vi "Create Plugins (old).vi"(5 "options":T1, 7 "framework configuration":T5, 8 "error in (no error)":errorcluster, 11 "Framework in":refnum<class "Framework.lvclass">) -> (0 "error out":errorcluster, 1 "Plugin Threads":refnum<class "Plugin Thread.lvclass">[](array[class]), 2 "Plugins":refnum<class "Plugin.lvclass">[](array[class]), 3 "Framework out":refnum<class "Framework.lvclass">)   [LabVIEW 2017, in "DSF Core.lvlib" / "Framework.lvclass"]
uses:
  Framework.lvclass
  Plugin/Plugin.lvclass
  DSF Configuration API/Public/Controls/DSF Engine Framework Configuration.ctl
  DSF Configuration API/Public/Controls/DSF Engine Plugin Configuration.ctl
  DSF Configuration API/Public/Controls/DSF Timing Info.ctl
  DSF Configuration API/Public/Controls/DSF Engine Transfer Group Configuration.ctl
  DSF Configuration API/Public/Controls/DSF Direction.ctl
  DSF Configuration API/Public/Controls/DSF Engine Transfer Configuration.ctl
  DSF Configuration API/Public/Controls/DSF Byte Order.ctl
  DSF Configuration API/Public/Controls/DSF Engine Channel Configuration.ctl
  DSF Configuration API/Public/Controls/DSF Data Type.ctl
  DSF Configuration API/Public/Controls/DSF Settings Info.ctl
  Thread/Plugin/Plugin Thread.lvclass
  Framework Options.ctl
  Typedefs/FIFO Flags.ctl
  Thread/Thread Options.ctl
  Typedefs/Plugin Flags.ctl
  Shared/VIs/Sizeof.vi
  DSF Configuration API/Public/Required Buffer Size (Plugin).vi
  DSF Configuration API/Public/Channel Count (Plugin).vi
  Component Loader/Component Loader.lvclass
  DSF Core.lvlib
  Buffer/Buffers.lvclass
  Buffer/Buffer.lvclass
  Thread/Thread.lvclass
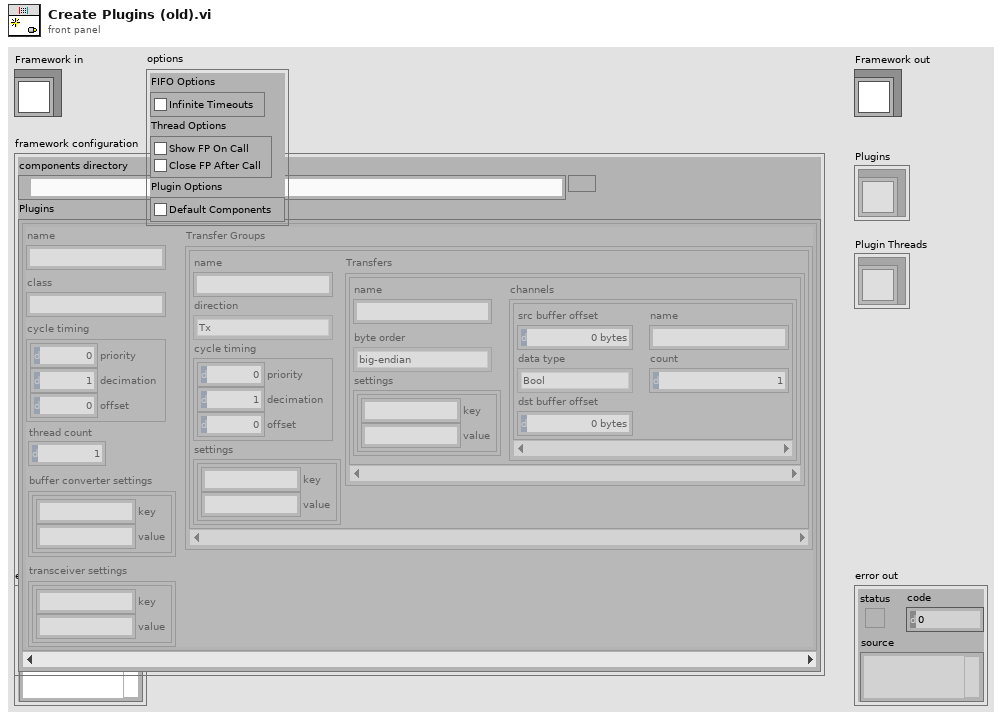
[diagram p1: front panel]
types:
  T1 = typedef "DSF Core.lvlib/Framework.lvclass/Framework Options.ctl" = cluster{"FIFO Options":T2, "Thread Options":T3, "Plugin Options":T4}
  T2 = typedef "DSF Core.lvlib/FIFO Flags.ctl" = cluster{"Infinite Timeouts":bool}
  T3 = typedef "DSF Core.lvlib/Thread.lvclass/Thread Options.ctl" = cluster{"Show FP On Call":bool, "Close FP After Call":bool}
  T4 = typedef "DSF Core.lvlib/Plugin Flags.ctl" = cluster{"Default Components":bool}
  T5 = typedef "DSF Core.lvlib/DSF Engine Framework Configuration.ctl" = cluster{"components directory":path, "Plugins":T6[]}
  T6 = typedef "DSF Core.lvlib/DSF Engine Plugin Configuration.ctl" = cluster{"name":string, "class":string, "cycle timing":T7, "Transfer Groups":T8[], "thread count":i32, "buffer converter settings":T14, "transceiver settings":T14}
  T7 = typedef "DSF Core.lvlib/DSF Timing Info.ctl" = cluster{"priority":u64, "decimation":u64, "offset":u64}
  T8 = typedef "DSF Core.lvlib/DSF Engine Transfer Group Configuration.ctl" = cluster{"name":string, "direction":T9, "cycle timing":T7, "Transfers":T10[], "settings":T14}
  T9 = typedef "DSF Core.lvlib/DSF Direction.ctl" = enum8{"Tx", "Rx"}
  T10 = typedef "DSF Core.lvlib/DSF Engine Transfer Configuration.ctl" = cluster{"name":string, "byte order":T11, "channels":T12[], "settings":T14}
  T11 = typedef "DSF Core.lvlib/DSF Byte Order.ctl" = enum8{"big-endian", "little-endian"}
  T12 = typedef "DSF Core.lvlib/DSF Engine Channel Configuration.ctl" = cluster{"src buffer offset":u64, "name":string, "data type":T13, "count":u64, "dst buffer offset":u64}
  T13 = typedef "DSF Core.lvlib/DSF Data Type.ctl" = enum8{"Bool", "SGL", "DBL", "I8", "I16", "I32", "I64", "U8", "U16", "U32", "U64"}
  T14 = typedef "DSF Core.lvlib/DSF Settings Info.ctl" = cluster{"key":string, "value":string}[]
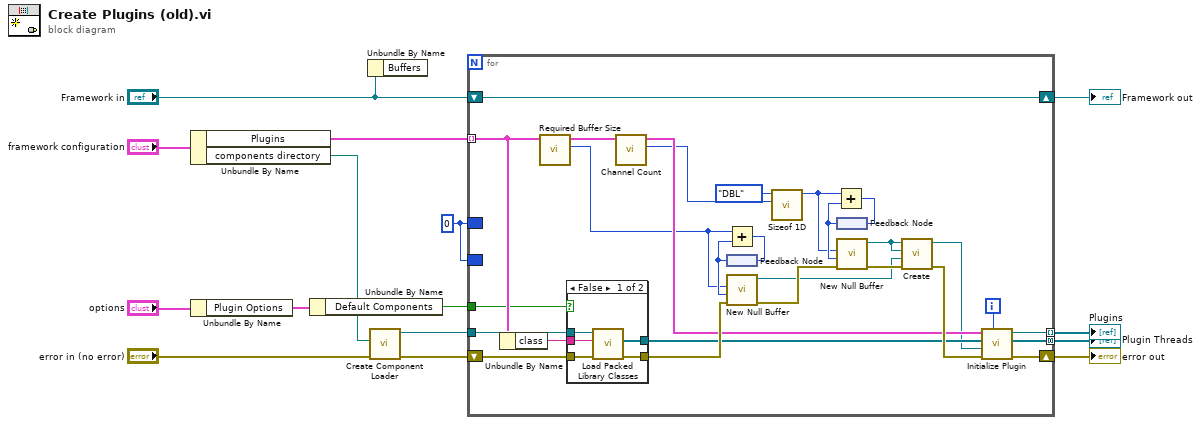
[diagram p0: block diagram]
diagram:
  w1 = u64 0 ("string buffer offset + size")
  n1 = Unbundle By Name("framework configuration") -> ("Plugins"=w9:T6[], "components directory"=w5:path)
  n2 = Unbundle By Name("options") -> ("Plugin Options"=w3:T4)
  n3 = Unbundle By Name(w3) -> ("Default Components"=w2:bool)
  n4 = Unbundle By Name("Framework in") -> ()  [unwired: 1 out]
  n5 = call "Create Component Loader.vi"("error in (no error)"="error in (no error)", "components directory (default)"=w5) -> ("error out"=w14:errorcluster, "Component Loader out"=w15:refnum<class "Component Loader.lvclass">)  [unwired: 8 in]
  n6 = for {
    shift-right: [w40] -> w11
    shift-left: w14 -> [w42]
    shift-right: [w25] -> w12
    shift-left: "Framework in" -> [w25]
    tunnel: w9 -> [w36] mode=indexing
    tunnel: w15 -> [w43]
    tunnel: [w39] -> w8 mode=indexing
    tunnel: [w38] -> w7 mode=concatenating
    border: w1 -> [_]
    border: w1 -> [_]
    tunnel: w2 -> [w34]
    i -> [w37]
    n7 = Unbundle By Name(w36) -> ("class"=w41:string)
    n8 = call-poly "Required Buffer Size.vi"("Plugin Configuration in"=w36) -> ("required buffer size"=w16:u64, "Plugin Configuration out"=w35:T6)  [unwired: 8 in, 1 out]
    n9 = case shown="False" w34 {
      tunnel: [w48 w49] -> w22
      tunnel: w43 -> [w47 _]
      tunnel: w42 -> [w46 w49]
      tunnel: w41 -> [w45 _]
      tunnel: [w44 _] -> w19
      frame False {
        n10 = call "Load Packed Library Classes.vi"("error in (no error)"=w46, "packed library name"=w45, "Component Loader in"=w47) -> ("error out"=w48:errorcluster, "objects"=w44:refnum<class>[])  [unwired: 6 in, 1 out]
      }
      frame True {
      }
    }
    n11 = call-poly "Channel Count.vi"("Plugin Configuration in"=w35) -> ("total channel count"=w17:u64, "Plugin Configuration out"=w20:T6)  [unwired: 8 in, 1 out]
    n12 = feedback #1() -> (w23:u64)
    n13 = Add(x=w16, y=w23) -> (x+y=w24:u64)
    n14 = feedback-in #1(w24) -> ()
    n15 = call "New Null Buffer.vi"("error in (no error)"=w22, "buffer offset"=w23, "buffer size"=w16) -> ("error out"=w30:errorcluster, "Buffer out"=w29:refnum<class "Buffer.lvclass">)  [unwired: 7 in]
    n16 = call "Sizeof 1D.vi"("count"=w17, "data type"=DSF_Data_Type."DBL") -> ("size in bytes"=w21:u64)  [unwired: 9 in]
    n17 = feedback #2() -> (w26:u64)
    n18 = Add(x=w21, y=w26) -> (x+y=w27:u64)
    n19 = feedback-in #2(w27) -> ()
    n20 = call "New Null Buffer.vi"("error in (no error)"=w30, "buffer offset"=w26, "buffer size"=w21) -> ("error out"=w32:errorcluster, "Buffer out"=w33:refnum<class "Buffer.lvclass">)  [unwired: 7 in]
    n21 = call "Create.vi"("error in (no error)"=w32, "String Buffer (null)"=w29, "Async Buffer (null)"=w33, "Inline Buffer (null)"=w33) -> ("error out"=w28:errorcluster, "Buffers out"=w18:refnum<class "Buffers.lvclass">)  [unwired: 6 in]
    n22 = call "Initialize Plugin.vi"("id"=w37, "error in (no error)"=w28, "Plugin Buffers"=w18, "component objects"=w19, "Plugin Configuration"=w20) -> ("error out"=w40:errorcluster, "Plugin Threads"=w38:refnum<class "Plugin Thread.lvclass">[], "Plugin out"=w39:refnum<class "Plugin.lvclass">)  [unwired: 4 in]
  }
  "error out" <- w11
  "Framework out" <- w12
  "Plugins" <- w8
  "Plugin Threads" <- w7
